vi "Util_GetTime_U32.vi"(8 "error in (no error)":errorcluster) -> (0 "error out":errorcluster, 3 "FPGA_Time_LowWord_MicroSeconds":u32 format="%.0g")   [LabVIEW 2019, in "Trajectory_Library.lvlib"]
doc: "This subVI returns the low word of the FPGA continuously running elapsed time in microseconds.\n\nThis is an internal routine and should NOT be called directly by the end user. \n\nOn the RoboRIO this reads the high resolution FPGA time. The resolution, not accuracy, of the FPGA timer is 1 microsecond. The normal FPGA clock register (32 bits) rolls over approximately every 71 minutes. To significantly extend the rollover time,, this routine reads both the high and low FPGA clock registers. High/low register turnover read sequencing is dealt with by reading the high register twice, once before and once after the low register. If the values are different, the read is repeated to assure consistency between the high and low values. On a PC the standard operating system timer with 1 millisecond resolution is used. \n\nNOTES:\n--------\n\n- Set a conditional complilation variable TRAJLIB_USEOSTIME and set it to a value of 1 to force this routine to read the RoboRIO operating system time instead of the FPGA time. This will have 1 millisecond resolution. This routine executes faster, approx 1 microsecond.\n\n - On the RoboRIO there is some drift between the FPGA and operating system clocks. The drift isn't consistent, but appears to be approximately 20 milliseconds / hour. This isn't enough to be of concern.\n\n\nInput parameters:\n - Error In -- Error Data Cluster -- \n\nReturns:\n - FPGA_Time_LowWord_Microseconds -- UInt32 -- Low word of continuously running FPGA clock.\n - Output Error -- Output error cluster. An error will be returned if there are problems reading the FPGA or of the FPGA clock high register changes twice while reading the value.\n\nCustom Errors:\n - 8020 -- The upper FPGA time register changed during both attempts to read the FPGA time values. The returned time may not be valid."
uses:
  Trajectory_Library.lvlib
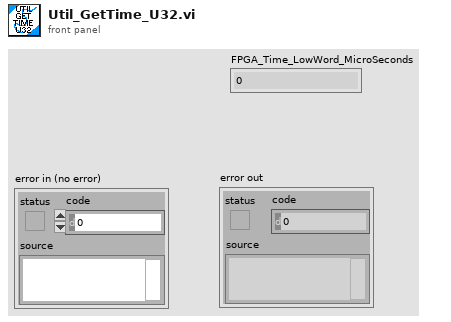
[diagram p1: front panel]
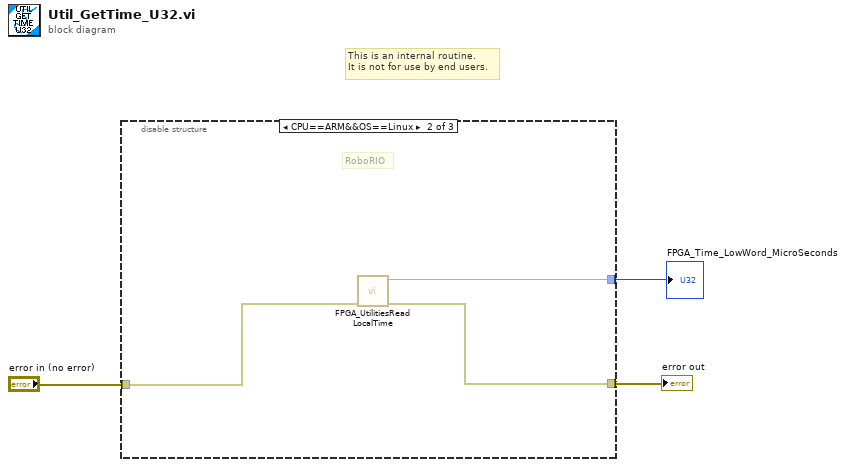
[diagram p0: block diagram]
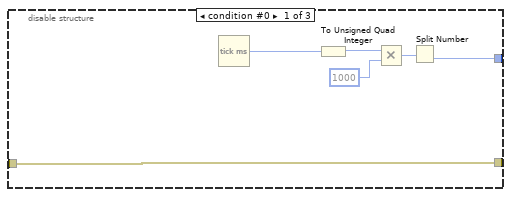
[diagram p2: hidden frame]
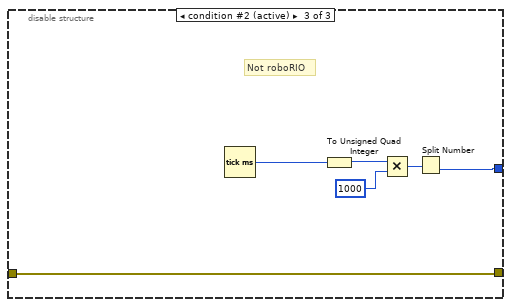
[diagram p3: hidden frame]
diagram:
  # "This is an internal routine.   \nIt is not for use by end users."
  n1 = disable-structure shown="CPU==ARM&&OS==Linux" {
    disable-tunnel: "error in (no error)" -> [w9 w10 w18]
    disable-tunnel: [w9 w11 w18] -> w2
    disable-tunnel: [w4 w12 w13] -> w1
    frame condition #0 {
      n2 = Tick Count (ms)() -> (millisecond timer value=w8:u32)
      n3 = To Unsigned Quad Integer(1:w8) -> (0:w7:u64)
      n4 = Multiply(x=w7, y=u64 1000) -> (x*y=w5:u64)
      n5 = Split Number(x=w5) -> (lo(x)=w4:u32)  [unwired: 1 out]
    }
    frame condition #1 {
      # "RoboRIO"
      n6 = call <vilib>:"FPGA_UtilitiesRead LocalTime.vi"("error in (no error)"=w10) -> ("error out"=w11:errorcluster, "LocalTime"=w12:u32)  [unwired: 9 out]
    }
    frame condition #2 (active) {
      # "Not roboRIO"
      n7 = Tick Count (ms)() -> (millisecond timer value=w17:u32)
      n8 = To Unsigned Quad Integer(1:w17) -> (0:w16:u64)
      n9 = Multiply(x=w16, y=u64 1000) -> (x*y=w14:u64)
      n10 = Split Number(x=w14) -> (lo(x)=w13:u32)  [unwired: 1 out]
    }
  }
  "error out" <- w2
  "FPGA_Time_LowWord_MicroSeconds" <- w1
